vi "FlatToRichni_measurementlink_sessionmanagement_v1_GetSessionsRequest.vi"(5 "OutputClusterType":T1, 11 "InputCluster":T2) -> (3 "OutputCluster":T1)   [LabVIEW 2021, in "ni.measurementlink.sessionmanagement.v1.api.lvlib"]
uses:
  ni.measurementlink.sessionmanagement.v1.api.lvlib
  ni_measurementlink_sessionmanagement_v1_GetSessionsRequest_Flat.ctl
  ni_measurementlink_sessionmanagement_v1_GetSessionsRequest.ctl
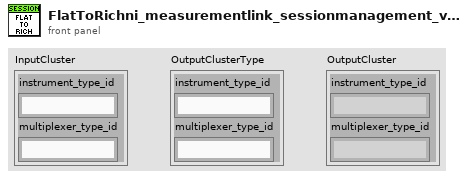
[diagram p1: front panel]
types:
  T1 = typedef "ni.measurementlink.sessionmanagement.v1.api.lvlib/ni_measurementlink_sessionmanagement_v1_GetSessionsRequest.ctl" = cluster{"instrument_type_id":string, "multiplexer_type_id":string}
  T2 = typedef "ni.measurementlink.sessionmanagement.v1.api.lvlib/ni_measurementlink_sessionmanagement_v1_GetSessionsRequest_Flat.ctl" = cluster{"instrument_type_id":string, "multiplexer_type_id":string}
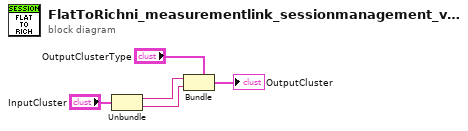
[diagram p0: block diagram]
diagram:
  n1 = Unbundle "Unbundle"("InputCluster") -> ("instrument_type_id"=w2:string, "multiplexer_type_id"=w1:string)
  n2 = Bundle "Bundle"(cluster="OutputClusterType", "instrument_type_id"=w2, "multiplexer_type_id"=w1) -> (→"OutputCluster":T1)
